vi "Startup_CheckUniFolder.vi"(7 "element":string, 8 "error in":errorcluster, 11 "path":path) -> (0 "error out":errorcluster, 3 "created path":path)   [LabVIEW 2016]
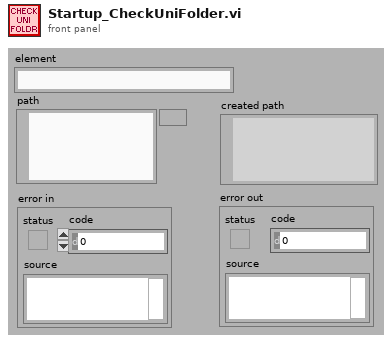
[diagram p1: front panel]
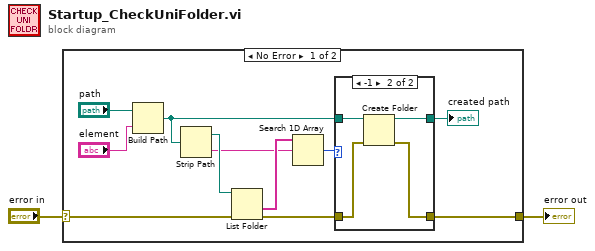
[diagram p0: block diagram]
diagram:
  n1 = case shown="No Error" "error in" {
    selector: "error in" -> [w8 w20]
    tunnel: [w10 w20] -> w2
    frame No Error {
      n2 = Build Path(base path="path", name or relative path="element") -> (appended path=w5:path)
      n3 = Strip Path(path=w5) -> (stripped path=w4:path, name=w3:string)
      n4 = List Folder(path=w4, error in=w8) -> (folder names=w13:string[], error out=w11:errorcluster)  [unwired: 4 out]
      n5 = Search 1D Array(1D array=w13, element=w3) -> (index of element=w12:i32)  [unwired: 1 out]
      n6 = case shown="-1" w12 {
        tunnel: w5 -> [w14 w16]
        tunnel: w11 -> [w15 w19]
        tunnel: [w14 w18] -> w9
        tunnel: [w15 w17] -> w10
        frame 0, Default {
        }
        frame -1 {
          n7 = Create Folder(path (use dialog)=w16, error in=w19) -> (created path=w18:path, error out=w17:errorcluster)  [unwired: 2 out]
        }
      }
      "created path" <- w9
    }
    frame Error {
    }
  }
  "error out" <- w2
